vi "Pump_Control.vi"(11 "Water Level":dbl) -> (2 "Pump 2 ON":bool, 3 "Pump 1 ON":bool)   [LabVIEW 2022 SP3]
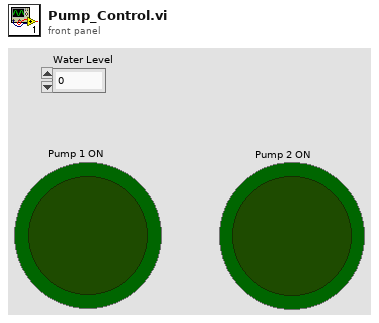
[diagram p1: front panel]
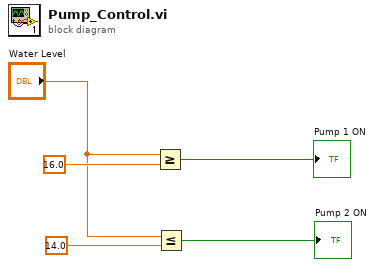
[diagram p0: block diagram]
diagram:
  n1 = Greater Or Equal?(x="Water Level", y=16.0) -> (x >= y?=→"Pump 1 ON":bool)
  n2 = Less Or Equal?(x="Water Level", y=14.0) -> (x <= y?=→"Pump 2 ON":bool)
